vi "SetSystemTimeZone_ZoneName.vi"(0 "Requested Timezone Name":string, 11 "Error in":errorcluster caption="Error in (no error)") -> (4 "UTC Offset Set":dbl, 15 "Error out":errorcluster)   [LabVIEW 2017, in "GPTiming.lvlib"]
doc: "Sets the <B>Requested Timezone Name</B> on the (Windows only) system.\n\n<B>Requested Timezone Name</B> must be one of the names available on the system, and thus present in the 'System Timezone Names' output of the GetSystemTimeZones VI.\n\nThe actual <B>UTC Offset Set</B> is returned.\n\nThis VI runs only if there is no error on <B>Error in</B>.\n\nSteen Schmidt\nGPower\n4/2 2017"
uses:
  GPTiming.lvlib
  Error/GPError.lvlib
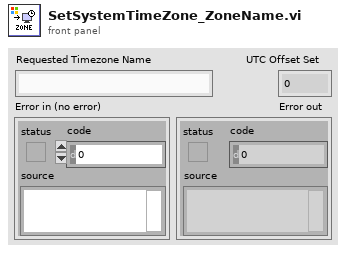
[diagram p1: front panel]
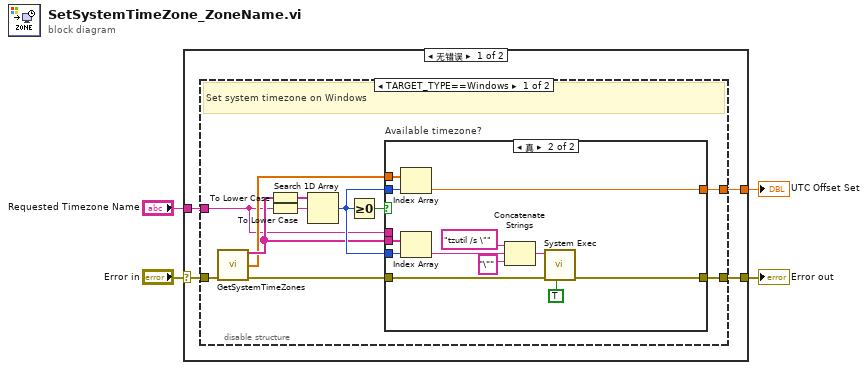
[diagram p0: block diagram]
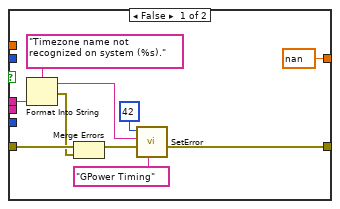
[diagram p2: hidden frame]
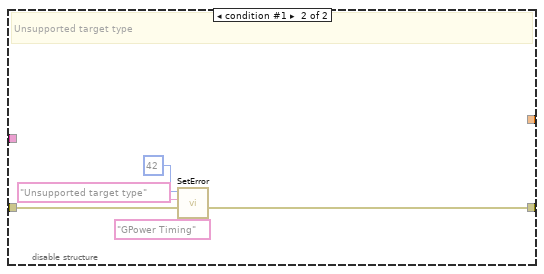
[diagram p3: hidden frame]
diagram:
  n1 = case shown="无错误" "Error in" {
    selector: "Error in" -> [w8 w47]
    tunnel: [w7 w47] -> w2
    tunnel: "Requested Timezone Name" -> [w6 _]
    tunnel: [w5 _] -> w1
    frame No Error {
      n2 = disable-structure shown="TARGET_TYPE==Windows" {
        disable-tunnel: w8 -> [w12 w44]
        disable-tunnel: [w11 w42] -> w7
        disable-tunnel: w6 -> [w10 _]
        disable-tunnel: [w9 _] -> w5
        frame condition #0 (active) {
          # "Set system timezone on Windows"
          n3 = call "GetSystemTimeZones.vi"("Error in"=w12) -> ("System Timezone Names"=w18:string[], "UTC Offsets"=w15:dbl[], "Error out"=w13:errorcluster)  [unwired: 11 in, 1 out]
          n4 = To Lower Case(string=w18) -> (all lower case string=w17:string[])
          n5 = To Lower Case(string=w10) -> (all lower case string=w16:string)
          n6 = Search 1D Array(1D array=w17, element=w16) -> (index of element=w19:i32)  [unwired: 1 in]
          n7 = Greater Or Equal To 0?(x=w19) -> (x >= 0?=w14:bool)
          n8 = case "Available timezone?" shown="真" w14 {
            tunnel: [w23 w41] -> w11
            tunnel: w13 -> [w28 w40]
            tunnel: w19 -> [_ w33]
            tunnel: w15 -> [_ w35]
            tunnel: [nan ("UTC offset") w34] -> w9
            tunnel: w10 -> [w25 _]
            tunnel: w18 -> [_ w32]
            tunnel: w19 -> [_ w31]
            frame False {
              n9 = Format Into String(format string="Timezone name not recognized on system (%s).", w25) -> (resulting string=w21:string, error out=w26:errorcluster)  [unwired: 2 in]
              n10 = Merge Errors(w28, w26) -> (w24:errorcluster)
              n11 = call "SetError.vi"("Error label"="GPower Timing", "Error in"=w24, "Error description"=w21, "Error code"=42) -> ("Error out"=w23:errorcluster)  [unwired: 7 in]
            }
            frame True {
              n12 = Index Array(array=w35, index=w33) -> (element=w34:dbl)
              n13 = Index Array(array=w32, index=w31) -> (element=w30:string)
              n14 = Concatenate Strings("tzutil /s \"" ("command line"), w30, "\"" ("command line")) -> (w36:string)
              n15 = call <vilib>:"System Exec.vi"("run minimized? (F)"=TRUE, "error in (no error)"=w40, "command line"=w36) -> ("error out"=w41:errorcluster)  [unwired: 5 in, 3 out]
            }
          }
        }
        frame condition #1 {
          # "Unsupported target type"
          n16 = call "SetError.vi"("Error label"="GPower Timing", "Error in"=w44, "Error description"="Unsupported target type", "Error code"=42) -> ("Error out"=w42:errorcluster)  [unwired: 7 in]
        }
      }
    }
    frame Error {
    }
  }
  "Error out" <- w2
  "UTC Offset Set" <- w1
